vi "PH_TKTDS-30xx.set initial i Attributes.vi"(2 "error in":errorcluster, 3 "Instance":string) -> (0 "error out":errorcluster, 1 "i Attri":T1={"Default VISA Resource"="N/A", "VISA Resource Name"="GPIB0::1::INSTR", "Revision"={"Instrument Driver"="", "Instrument Firmware"=""}, "Selftest"={"Result"=0, "Message"="N/A"}, "Channels"=[], "Trigger Configuration"={"Source"="CH1", "Slope"=0, "Level [V]"=0.0}, "Acquisition Configuration"={"Time base"=2e-07, "Record Length"=10000, "Start Time"=0.0, "Type"=0, "Continuous"=FALSE}, "Fetched Waveforms"=[], "GUI Refs"={"Trigger"=refnum, "Acquisition"=refnum, "Graph"=refnum, "State"=refnum, "Delete"=refnum, "Channel to be positioned"=refnum, "Postion"=refnum, "Display Intensity"=refnum, "VISA Resource"=refnum}, "GUI Refs Channels"=[], "State"=0, "Error Message"="", "Allow Prdc Loop?"=FALSE} {"State" items=["no info", "off/false/out", "on/true/in", "Failure", "Alarm", "Status 1", "Status 2", "Status 3"]; "Fetched Waveforms"."Waveform Array" format="%.2f"; "Fetched Waveforms"."X Increment" format="%.2e"; "Fetched Waveforms"."Initial X" format="%.2e"; "Acquisition Configuration"."Start Time" format="%#_12p"; "Acquisition Configuration"."Record Length" items=["500"=500, "10000"=10000]; "Acquisition Configuration"."Time base" items=["2ns"=2e-09, "4ns"=4e-09, "10ns"=1e-08, "20ns"=2e-08, "40ns"=4e-08, "100ns"=1e-07, "200ns"=2e-07, "400ns"=4e-07, "1µs"=1e-06, "2µs"=2e-06, "4µs"=4e-06, "10µs"=1e-05, "20µs"=2e-05, "40µs"=4e-05, "100µs"=0.0001, "200µs"=0.0002, "400µs"=0.0004, "1ms"=0.001, "2ms"=0.002, "10ms"=0.01, "20ms"=0.02, "40ms"=0.04, "100ms"=0.1, "200ms"=0.2, "400ms"=0.4, "1s"=1.0, "2s"=2.0, "4s"=4.0, "10s"=10.0]; "Trigger Configuration"."Level [V]" format="%#_6p"; "Channels"."Vertical Offset" format="%#_6p"; "Channels"."Vertical Range" items=["1mV"=0.001, "2mV"=0.002, "5mV"=0.005, "10mV"=0.01, "20mV"=0.02, "50mV"=0.05, "100mV"=0.1, "200mV"=0.2, "500mV"=0.5, "1V"=1.0]; "Channels"."Probe Attenuation" format="%#.2f"; "Selftest"."Result" format="%.0x"})   [LabVIEW 2014, in "PH_TKTDS-30xx.lvlib"]
doc: "This VI sets Attributes to a default state."
uses:
  PH_TKTDS-30xx.lvlib
  PH_TKTDS-30xx.i attribute.ctl
  PH_TKTDS-30xx.Channel Config.ctl
  PH_TKTDS-30xx.Trigger Config.ctl
  PH_TKTDS-30xx.Acquisition Config.ctl
  PH_TKTDS-30xx.fetched Waveform.ctl
  PH_TKTDS-30xx.GUI Refs.ctl
  PH_StatusHandler/PH_StatusHandler.Status.ctl
  PH_StatusHandler/PH_StatusHandler.lvlib
  PH_Common/PH_Common.lvlib
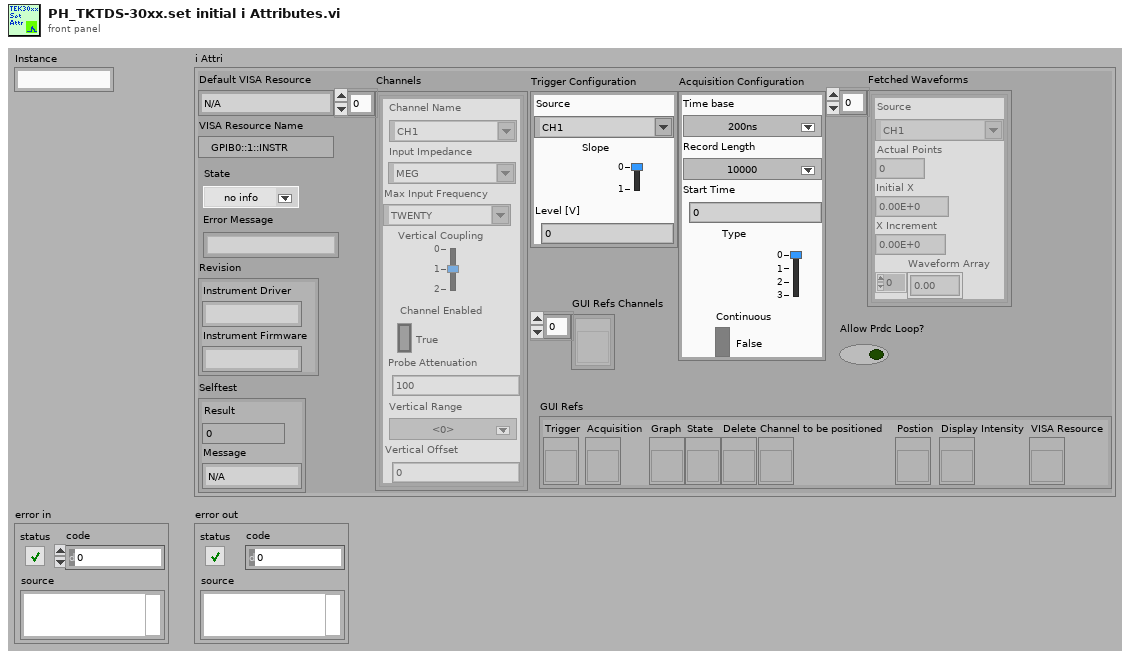
[diagram p1: front panel]
types:
  T1 = typedef "PH_TKTDS-30xx.lvlib/PH_TKTDS-30xx.i attribute.ctl" = cluster{"Default VISA Resource":string, "VISA Resource Name":refnum<visa-resource-name>, "Revision":cluster{"Instrument Driver":string, "Instrument Firmware":string}, "Selftest":cluster{"Result":u32, "Message":string}, "Channels":T2[], "Trigger Configuration":T3, "Acquisition Configuration":T4, "Fetched Waveforms":T5[], "GUI Refs":T6, "GUI Refs Channels":refnum<vi>[], "State":T7, "Error Message":string, "Allow Prdc Loop?":bool}
  T2 = typedef "PH_TKTDS-30xx.lvlib/PH_TKTDS-30xx.Channel Config.ctl" = cluster{"Channel Name":string, "Input Impedance":string, "Max Input Frequency":string, "Vertical Coupling":i32, "Channel Enabled":bool, "Probe Attenuation":dbl, "Vertical Range":dbl, "Vertical Offset":dbl}
  T3 = typedef "PH_TKTDS-30xx.lvlib/PH_TKTDS-30xx.Trigger Config.ctl" = cluster{"Source":string, "Slope":i32, "Level [V]":dbl}
  T4 = typedef "PH_TKTDS-30xx.lvlib/PH_TKTDS-30xx.Acquisition Config.ctl" = cluster{"Time base":dbl, "Record Length":u16, "Start Time":dbl, "Type":i32, "Continuous":bool}
  T5 = typedef "PH_TKTDS-30xx.lvlib/PH_TKTDS-30xx.fetched Waveform.ctl" = cluster{"Source":string, "Actual Points":u32, "Initial X":dbl, "X Increment":dbl, "Waveform Array":dbl[]}
  T6 = typedef "PH_TKTDS-30xx.lvlib/PH_TKTDS-30xx.GUI Refs.ctl" = cluster{"Trigger":refnum<vi>, "Acquisition":refnum<vi>, "Graph":refnum<vi>, "State":refnum<vi>, "Delete":refnum<vi>, "Channel to be positioned":refnum<vi>, "Postion":refnum<vi>, "Display Intensity":refnum<vi>, "VISA Resource":refnum<vi>}
  T7 = typedef "PH_StatusHandler.lvlib/PH_StatusHandler.Status.ctl" = i16
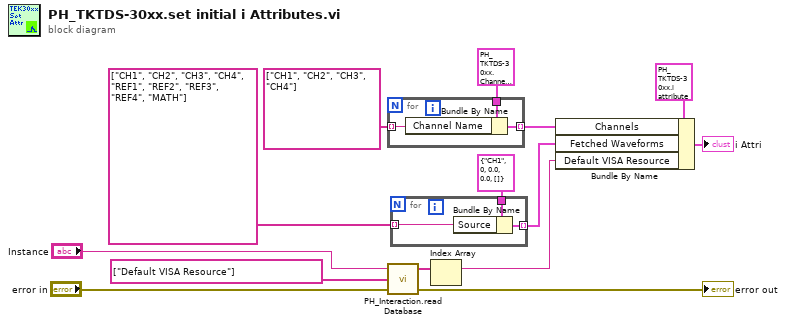
[diagram p0: block diagram]
diagram:
  n1 = for {
    tunnel: T2 {"Channel Name"="CH1", "Input Impedance"="MEG", "Max Input Frequency"="TWENTY", "Vertical Coupling"=1, "Channel Enabled"=TRUE, "Probe Attenuation"=0.1, "Vertical Range"=0.0, "Vertical Offset"=0.0} ("Channel Configuration") -> [w17]
    tunnel: string[] ["CH1", "CH2", "CH3", "CH4"] -> [w16] mode=indexing
    tunnel: [w15] -> w12 mode=indexing
    n2 = Bundle By Name(cluster=w17, "Channel Name"=w16) -> (w15:T2)
  }
  n3 = call "PH_Interaction.read Database.vi"("error in (no error)"="error in", "Strings to search for"=string[] ["Default VISA Resource"] ("Strings to search for in"), "DB Entry to read"="Instance") -> ("error out"=→"error out":errorcluster, "Values"=w2:string[])  [unwired: 1 in]
  n4 = for {
    tunnel: T5 {"Source"="CH1", "Actual Points"=0, "Initial X"=0.0, "X Increment"=0.0, "Waveform Array"=[]} ("Fetched Waveform") -> [w20]
    tunnel: string[] ["CH1", "CH2", "CH3", "CH4", "REF1", "REF2", "REF3", "REF4", "MATH"] -> [w19] mode=indexing
    tunnel: [w18] -> w9 mode=indexing
    n5 = Bundle By Name(cluster=w20, "Source"=w19) -> (w18:T5)
  }
  n6 = Index Array(array=w2) -> (element=w1:string)  [unwired: 1 in]
  n7 = Bundle By Name(cluster=T1 {"Default VISA Resource"="N/A", "VISA Resource Name"="GPIB0::1::INSTR", "Revision"={"Instrument Driver"="", "Instrument Firmware"=""}, "Selftest"={"Result"=0, "Message"="N/A"}, "Channels"=[], "Trigger Configuration"={"Source"="CH1", "Slope"=0, "Level [V]"=0.0}, "Acquisition Configuration"={"Time base"=2e-07, "Record Length"=10000, "Start Time"=0.0, "Type"=0, "Continuous"=FALSE}, "Fetched Waveforms"=[], "GUI Refs"={"Trigger"=refnum, "Acquisition"=refnum, "Graph"=refnum, "State"=refnum, "Delete"=refnum, "Channel to be positioned"=refnum, "Postion"=refnum, "Display Intensity"=refnum, "VISA Resource"=refnum}, "GUI Refs Channels"=[], "State"=0, "Error Message"="", "Allow Prdc Loop?"=FALSE} ("i Attri"), "Channels"=w12, "Fetched Waveforms"=w9, "Default VISA Resource"=w1) -> (→"i Attri":T1)
